vi "Get zoom factor based parameters.vi"(9 "Small FOV?":bool, 10 "Zoom factor\nprevious iteration\nvalue in":dbl, 11 "Zoom factor\ncompare":dbl) -> (1 "Apply overlay?":bool, 2 "Zoom factor\nprevious iteration\nvalue":dbl, 3 "Overlay variations":T1)   [LabVIEW 2019]
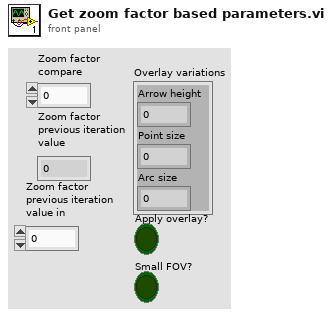
[diagram p1: front panel]
types:
  T1 = cluster{"Arrow height":dbl, "Point size":dbl, "Arc size":dbl}
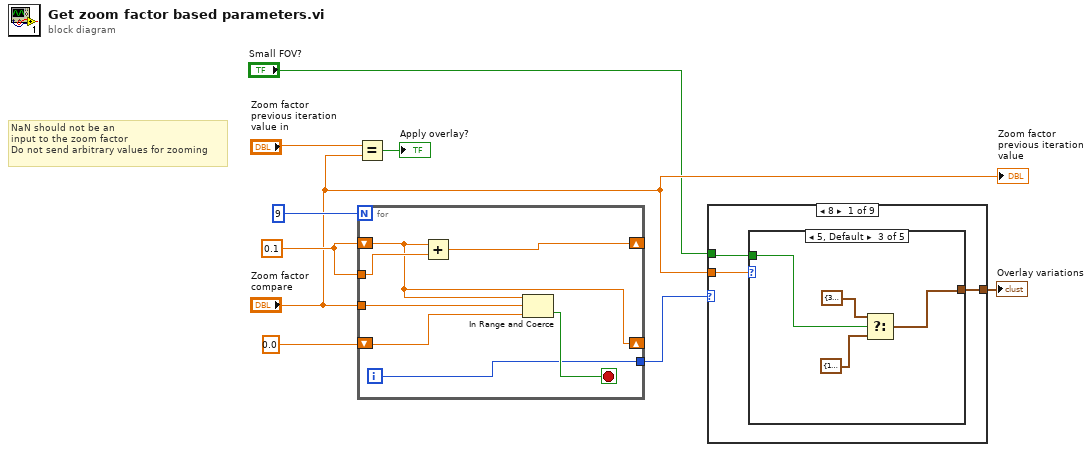
[diagram p0: block diagram]
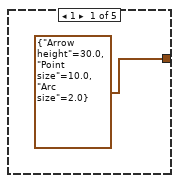
[diagram p2: hidden frame]
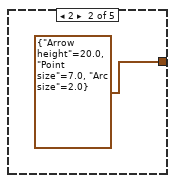
[diagram p3: hidden frame]
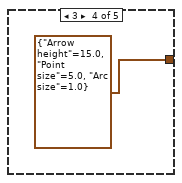
[diagram p4: hidden frame]
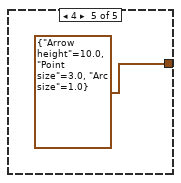
[diagram p5: hidden frame]
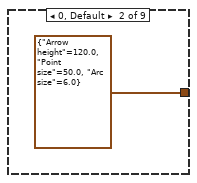
[diagram p6: hidden frame]
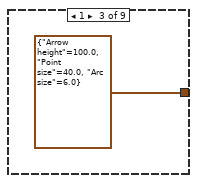
[diagram p7: hidden frame]
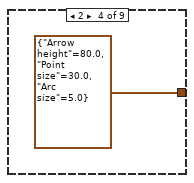
[diagram p8: hidden frame]
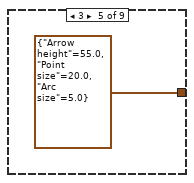
[diagram p9: hidden frame]
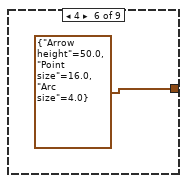
[diagram p10: hidden frame]
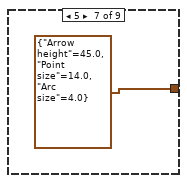
[diagram p11: hidden frame]
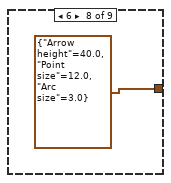
[diagram p12: hidden frame]
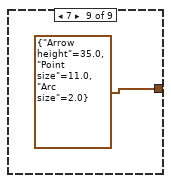
[diagram p13: hidden frame]
diagram:
  w8 = 0.1 ("upper limit")
  # "NaN should not be an \ninput to the zoom factor\nDo not send arbitrary values for zooming"
  n1 = Equal?(x="Zoom factor\nprevious iteration\nvalue in", y="Zoom factor\ncompare") -> (x = y?=→"Apply overlay?":bool)
  n2 = for {
    N: 9 -> [_]
    tunnel: "Zoom factor\ncompare" -> [w16]
    tunnel: w8 -> [w13]
    shift-right: [w10] -> _
    shift-left: 0.0 ("lower limit") -> [w15]
    shift-right: [w14] -> _
    shift-left: w8 -> [w10]
    tunnel: [w11] -> w6
    i -> [w11]
    stop <- w12 stop-if-true
    n3 = Add(x=w10, y=w13) -> (x+y=w14:dbl)
    n4 = In Range and Coerce(upper limit=w10, x=w16, lower limit=w15) -> (In Range?=w12:bool)  [unwired: 1 out]
  }
  n5 = case shown="8" w6 {
    tunnel: "Zoom factor\ncompare" -> [w19 _ _ _ _ _ _ _ _]
    tunnel: [w18 T1 {"Arrow height"=120.0, "Point size"=50.0, "Arc size"=6.0} ("Overlay variations") T1 {"Arrow height"=100.0, "Point size"=40.0, "Arc size"=6.0} ("Overlay variations") T1 {"Arrow height"=80.0, "Point size"=30.0, "Arc size"=5.0} ("Overlay variations") T1 {"Arrow height"=55.0, "Point size"=20.0, "Arc size"=5.0} ("Overlay variations") T1 {"Arrow height"=50.0, "Point size"=16.0, "Arc size"=4.0} ("Overlay variations") T1 {"Arrow height"=45.0, "Point size"=14.0, "Arc size"=4.0} ("Overlay variations") T1 {"Arrow height"=40.0, "Point size"=12.0, "Arc size"=3.0} ("Overlay variations") T1 {"Arrow height"=35.0, "Point size"=11.0, "Arc size"=2.0} ("Overlay variations")] -> w5
    tunnel: "Small FOV?" -> [w17 _ _ _ _ _ _ _ _]
    frame 8 {
      n6 = case shown="5, Default" w19 {
        tunnel: [T1 {"Arrow height"=30.0, "Point size"=10.0, "Arc size"=2.0} ("Overlay variations") T1 {"Arrow height"=20.0, "Point size"=7.0, "Arc size"=2.0} ("Overlay variations") w22 T1 {"Arrow height"=15.0, "Point size"=5.0, "Arc size"=1.0} ("Overlay variations") T1 {"Arrow height"=10.0, "Point size"=3.0, "Arc size"=1.0} ("Overlay variations")] -> w18
        tunnel: w17 -> [_ _ w23 _ _]
        frame 1 {
        }
        frame 2 {
        }
        frame 5, Default {
          n7 = Select(t=T1 {"Arrow height"=35.0, "Point size"=3.0, "Arc size"=1.5} ("Overlay variations"), s=w23, f=T1 {"Arrow height"=10.0, "Point size"=3.0, "Arc size"=1.0} ("Overlay variations")) -> (s? t:f=w22:T1)
        }
        frame 3 {
        }
        frame 4 {
        }
      }
    }
    frame 0, Default {
    }
    frame 1 {
    }
    frame 2 {
    }
    frame 3 {
    }
    frame 4 {
    }
    frame 5 {
    }
    frame 6 {
    }
    frame 7 {
    }
  }
  "Overlay variations" <- w5
  "Zoom factor\nprevious iteration\nvalue" <- "Zoom factor\ncompare"
